vi "S2C_FORNAX_Proc_ManageMsgSize.vi"(7 "Msg In":T1, 8 "Error In":errorcluster) -> (0 "Error Out":errorcluster, 5 "Msg Out":T1)   [LabVIEW 2015]
doc: "Keeps the ViperMsg and DDSMsg arrays to 1000 characters or less."
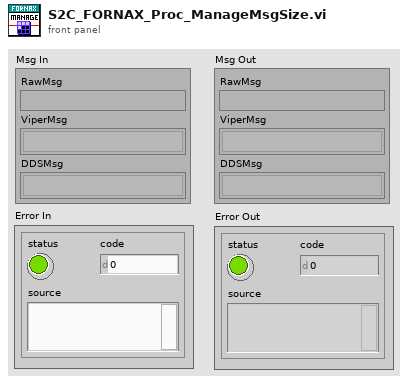
[diagram p1: front panel]
types:
  T1 = cluster{"RawMsg":string, "ViperMsg":string[], "DDSMsg":string[]}
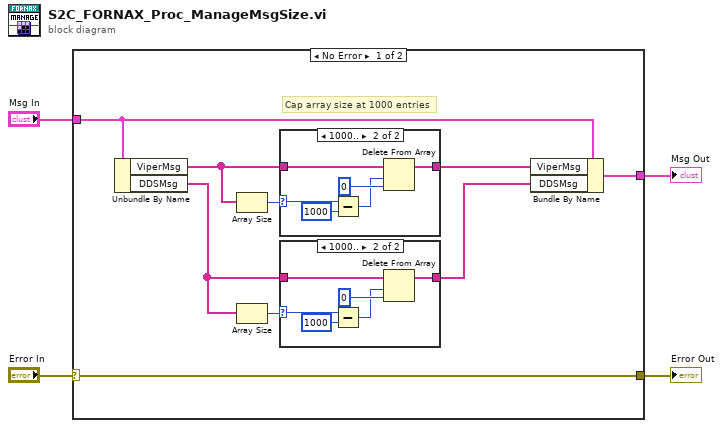
[diagram p0: block diagram]
diagram:
  n1 = case shown="No Error" "Error In" {
    selector: "Error In" -> [w5 w28]
    tunnel: "Msg In" -> [w13 w29]
    tunnel: [w6 w29] -> w3
    tunnel: [w5 w28] -> w1
    frame No Error {
      # "Cap array size at 1000 entries"
      n2 = Unbundle By Name(w13) -> ("ViperMsg"=w8:string[], "DDSMsg"=w11:string[])
      n3 = Array Size(array=w8) -> (size(s)=w9:i32)
      n4 = Array Size(array=w11) -> (size(s)=w12:i32)
      n5 = case shown="1000.." w9 {
        selector: w9 -> [_ w18]
        tunnel: w8 -> [w14 w20]
        tunnel: [w14 w15] -> w7
        frame 0, Default {
        }
        frame 1000.. {
          n6 = Subtract(x=w18, y=1000) -> (x-y=w16:i32)
          n7 = Delete From Array(array=w20, length=w16, index=0 ("dimension size")) -> (array with subset deleted=w15:string[])  [unwired: 1 out]
        }
      }
      n8 = case shown="1000.." w12 {
        selector: w12 -> [_ w25]
        tunnel: w11 -> [w21 w27]
        tunnel: [w21 w22] -> w10
        frame 0, Default {
        }
        frame 1000.. {
          n9 = Subtract(x=w25, y=1000) -> (x-y=w23:i32)
          n10 = Delete From Array(array=w27, length=w23, index=0 ("dimension size")) -> (array with subset deleted=w22:string[])  [unwired: 1 out]
        }
      }
      n11 = Bundle By Name(cluster=w13, "ViperMsg"=w7, "DDSMsg"=w10) -> (w6:T1)
    }
    frame Error {
    }
  }
  "Error Out" <- w1
  "Msg Out" <- w3
